vi "sub_ReadInput.vi"(8 "error in (no error)":errorcluster, 10 "Dynamic data":T1, 11 "Input parameters":T2={"Measurement type"=enum."Test", "Sensor type"=enum."HPK_8in_256", "Identifier"="test.txt", "Open after execution?"=FALSE, "Plot after execution?"=FALSE, "Display channel"=0, "Voltage Delay (s)"=0.5, "Switch Delay (s)"=0.01, "VISA resource name source"="", "VISA resource name DMM"="", "VISA resource name LCR"="", "Compliance  Level (uA)"=10.0, "Voltage Limit (V)"=1000.0, "Data storage location"="", "Scan voltages"="", "Use source as DMM?"=FALSE, "Single channel?"=FALSE, "LCR signal frequenzy (Hz)"=10.0} {"Voltage Limit (V)" format="%#_13g"; "Voltage Delay (s)" format="%#_13g"; "Switch Delay (s)" format="%#_13g"}) -> (0 "error out":errorcluster, 2 "Dynamic data":T1, 3 "Input parameters":T2={"Measurement type"=enum."Test", "Sensor type"=enum."HPK_8in_256", "Identifier"="test.txt", "Open after execution?"=FALSE, "Plot after execution?"=FALSE, "Display channel"=0, "Voltage Delay (s)"=0.5, "Switch Delay (s)"=0.01, "VISA resource name source"="", "VISA resource name DMM"="", "VISA resource name LCR"="", "Compliance  Level (uA)"=10.0, "Voltage Limit (V)"=1000.0, "Data storage location"="", "Scan voltages"="", "Use source as DMM?"=FALSE, "Single channel?"=FALSE, "LCR signal frequenzy (Hz)"=10.0} {"Voltage Limit (V)" format="%#_13g"; "Voltage Delay (s)" format="%#_13g"; "Switch Delay (s)" format="%#_13g"})   [LabVIEW 2016]
uses:
  Input_parameters.ctl
  Dynamic_data.ctl
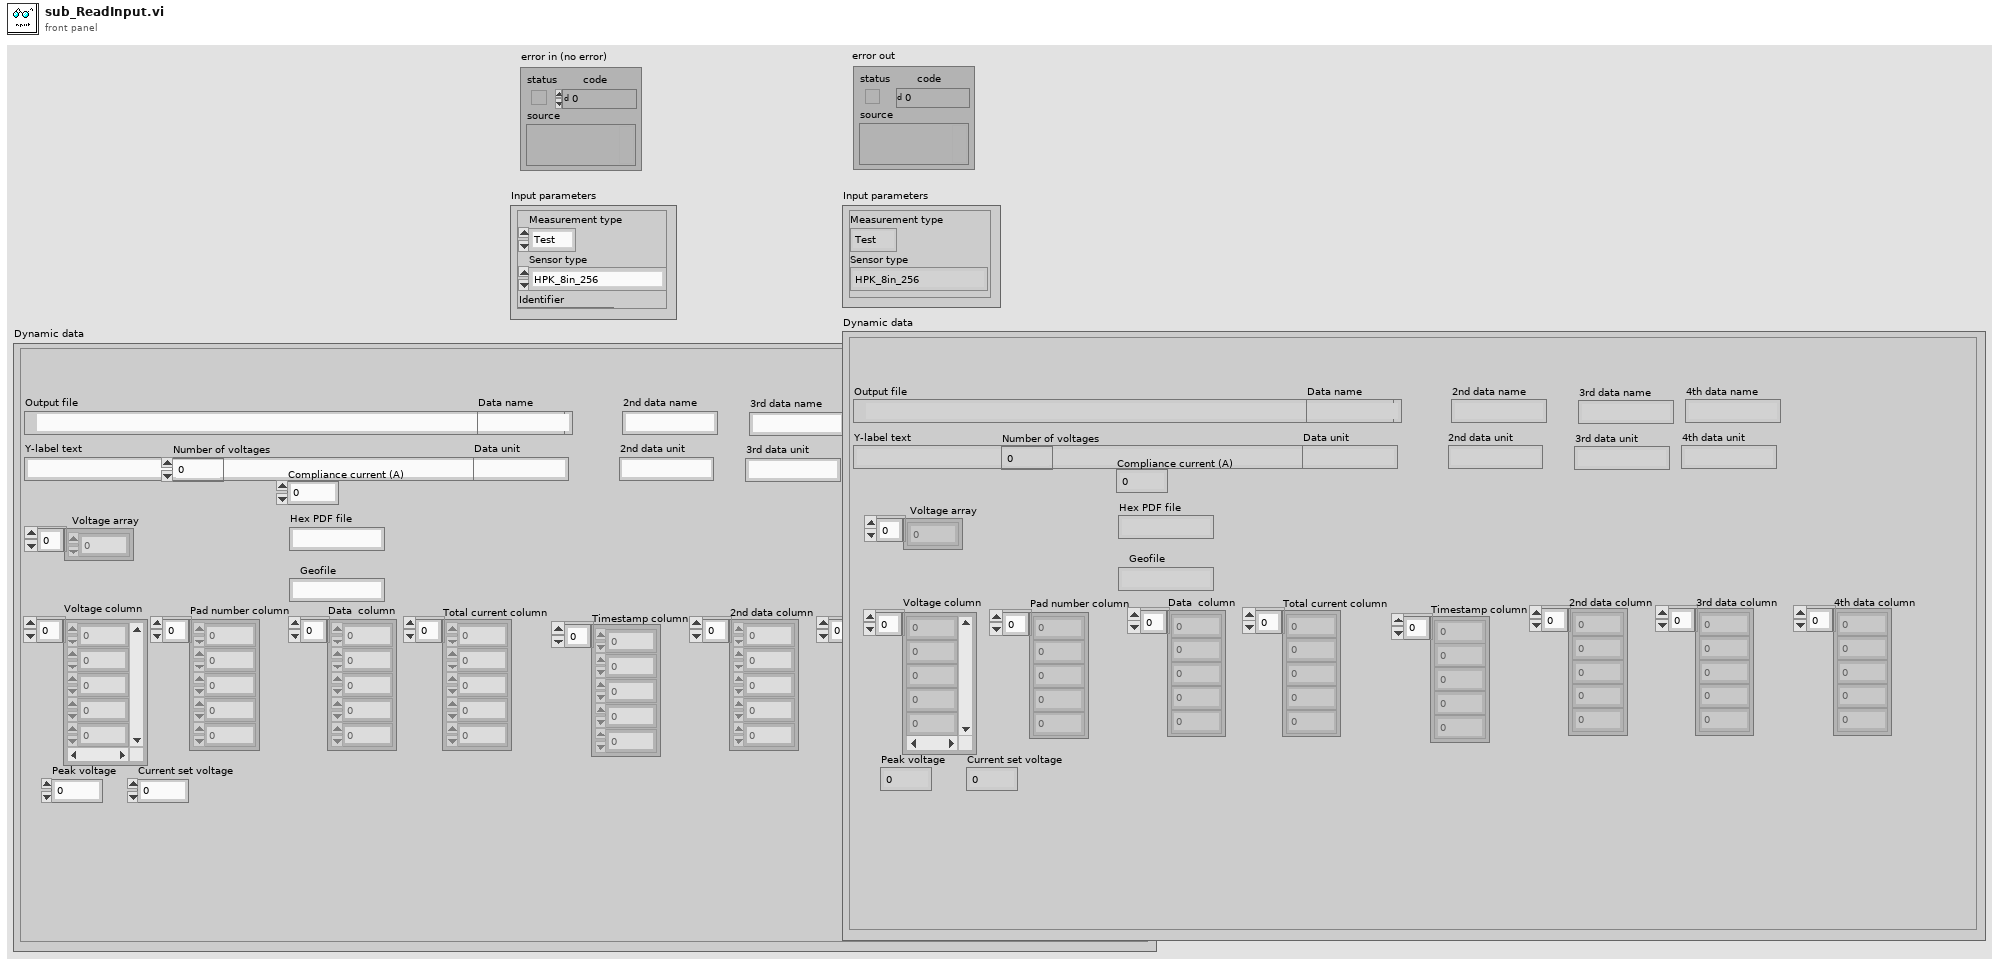
[diagram p1: front panel]
types:
  T1 = typedef "Dynamic_data.ctl" = cluster{"Output file":path, "Y-label text":string, "Current set voltage":dbl, "Voltage column":dbl[], "Pad number column":dbl[], "Data  column":dbl[], "Number of voltages":i32, "Compliance current (A)":dbl, "Geofile":string, "Peak voltage":dbl, "Hex PDF file":string, "Voltage array":dbl[], "Total current column":dbl[], "Timestamp column":dbl[], "Data name":string, "Data unit":string, "2nd data column":dbl[], "2nd data name":string, "2nd data unit":string, "3rd data column":dbl[], "4th data column":dbl[], "3rd data name":string, "3rd data unit":string, "4th data name":string, "4th data unit":string}
  T2 = typedef "Input_parameters.ctl" = cluster{"Measurement type":enum16{"IV", "CV", "Test"}, "Sensor type":enum16{"HPK_6in_135", "HPK_8in_256", "INF_8in_256", "Diode"}, "Identifier":string, "Open after execution?":bool, "Plot after execution?":bool, "Display channel":i32, "Voltage Delay (s)":dbl, "Switch Delay (s)":dbl, "VISA resource name source":refnum<visa-resource-name>, "VISA resource name DMM":refnum<visa-resource-name>, "VISA resource name LCR":refnum<visa-resource-name>, "Compliance  Level (uA)":dbl, "Voltage Limit (V)":dbl, "Data storage location":string, "Scan voltages":string, "Use source as DMM?":bool, "Single channel?":bool, "LCR signal frequenzy (Hz)":dbl}
  T3 = enum16{"HPK_6in_135", "HPK_8in_256", "INF_8in_256", "Diode"}
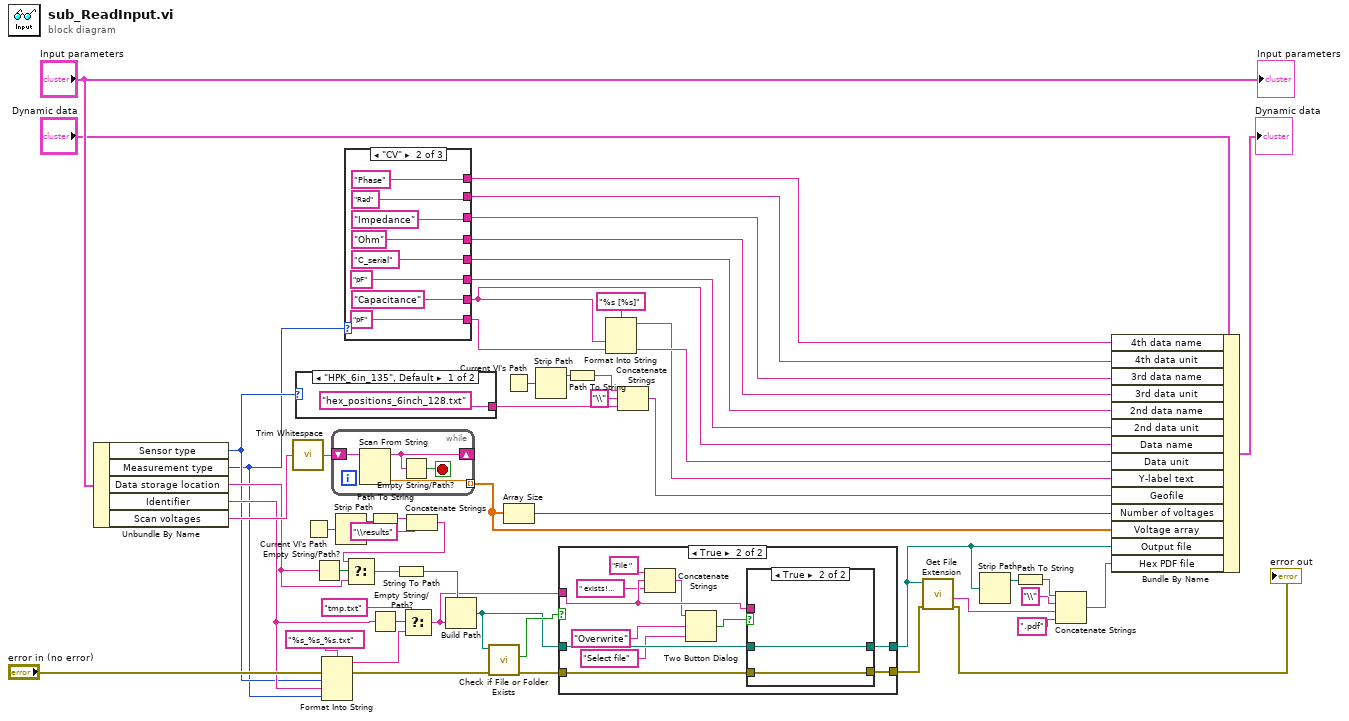
[diagram p0: block diagram]
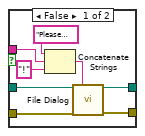
[diagram p3: hidden frame]
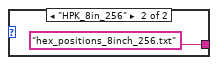
[diagram p4: hidden frame]
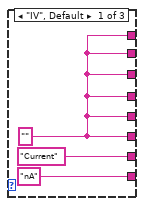
[diagram p5: hidden frame]
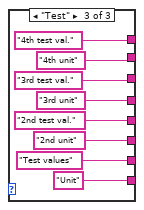
[diagram p6: hidden frame]
diagram:
  n1 = Unbundle By Name("Input parameters") -> ("Sensor type"=w20:T3, "Measurement type"=w19:enum16{"IV", "CV", "Test"}, "Data storage location"=w31:string, "Identifier"=w21:string, "Scan voltages"=w39:string)
  n2 = call <vilib>:"Trim Whitespace.vi"("string"=w39) -> ("trimmed string"=w40:string)  [unwired: 1 in]
  n3 = case shown="\"HPK_6in_135\", Default" w20 {
    tunnel: ["hex_positions_6inch_128.txt" "hex_positions_8inch_256.txt" ("name or relative path")] -> w51
    frame "HPK_6in_135", Default {
    }
    frame "HPK_8in_256" {
    }
  }
  n4 = Current VI's Path() -> (path=w35:path)
  n5 = Empty String/Path?(string/path=w31) -> (empty?=w36:bool)
  n6 = Format Into String(format string="%s_%s_%s.txt", error in="error in (no error)", w20, w21, w19) -> (resulting string=w23:string, error out=w13:errorcluster)  [unwired: 1 in]
  n7 = while {
    shift-right: [w58] -> _
    shift-left: w40 -> [w59]
    tunnel: [w60] -> w41 mode=indexing
    stop <- w57 stop-if-true
    n8 = Scan From String(input string=w59) -> (remaining string=w58:string, output 1=w60:dbl)  [unwired: 4 in, 2 out]
    n9 = Empty String/Path?(string/path=w58) -> (empty?=w57:bool)
  }
  n10 = Strip Path(path=w35) -> (stripped path=w34:path)  [unwired: 1 out]
  n11 = case shown="\"CV\"" w19 {
    tunnel: ["Current" "Capacitance" "Test values"] -> w9
    tunnel: ["nA" "pF" "Unit"] -> w10
    tunnel: [w61 "C_serial" "2nd test val."] -> w8
    tunnel: [w61 "pF" "2nd unit"] -> w7
    tunnel: [w61 "Ohm" "3rd unit"] -> w4
    tunnel: [w61 "Impedance" "3rd test val."] -> w3
    tunnel: [w61 "Rad" "4th unit"] -> w2
    tunnel: [w61 "Phase" "4th test val."] -> w1
    frame "IV", Default {
      w61 = ""
    }
    frame "CV" {
    }
    frame "Test" {
    }
  }
  n12 = Path To String(path=w34) -> (string=w33:string)
  n13 = Empty String/Path?(string/path=w21) -> (empty?=w27:bool)
  n14 = Select(t="tmp.txt", s=w27, f=w23) -> (s? t:f=w12:string)
  n15 = Concatenate Strings(w33, "\\results" ("string")) -> (w30:string)
  n16 = Select(t=w30, s=w36, f=w31) -> (s? t:f=w29:string)
  n17 = String To Path(string=w29) -> (path=w28:path)
  n18 = Build Path(base path=w28, name or relative path=w12) -> (appended path=w17:path)
  n19 = call <vilib>:"Check if File or Folder Exists.vi"("error in (no error)"=w13, "path"=w17) -> ("error out"=w15:errorcluster, "file or folder exists?"=w18:bool)  [unwired: 7 in, 1 out]
  n20 = Current VI's Path() -> (path=w38:path)
  n21 = Array Size(array=w41) -> (size(s)=w42:i32)
  n22 = Strip Path(path=w38) -> (stripped path=w37:path)  [unwired: 1 out]
  n23 = case shown="True" w18 {
    tunnel: w17 -> [w81 w92]
    tunnel: [w81 w91] -> w16
    tunnel: w15 -> [w80 w90]
    tunnel: [w80 w89] -> w14
    tunnel: w12 -> [_ w88]
    frame False {
    }
    frame True {
      n24 = Concatenate Strings("File " ("string"), w88, " exists! Overwite?" ("string")) -> (w85:string)
      n25 = Two Button Dialog(message=w85, 1:"Select file" ("Center Button Text (\"No\")"), 2:"Overwrite" ("Left Button Text (\"Yes\")")) -> (T button?=w82:bool)
      n26 = case shown="True" w82 {
        tunnel: w92 -> [w100 w102]
        tunnel: [w99 w102] -> w91
        tunnel: w90 -> [w98 w101]
        tunnel: [w97 w101] -> w89
        tunnel: w88 -> [w94 _]
        frame False {
          n27 = Concatenate Strings("Please chose a new file instead of  " ("prompt (Choose or enter file path)"), w94, "!" ("string")) -> (w96:string)
          n28 = call "File Dialog"("start path"=w100, "prompt"=w96, "error in"=w98) -> ("selected path"=w99:path, "error out"=w97:errorcluster)  [unwired: 9 in, 2 out]
        }
        frame True {
        }
      }
    }
  }
  n29 = Path To String(path=w37) -> (string=w25:string)
  n30 = Format Into String(format string="%s [%s]", w9, w10) -> (resulting string=w5:string)  [unwired: 2 in, 1 out]
  n31 = Concatenate Strings(w25, "\\" ("string"), w51) -> (w6:string)
  n32 = call <vilib>:"Get File Extension.vi"("error in (no error)"=w14, "file"=w16) -> ("error out"=→"error out":errorcluster, "filename without extension"=w48:string)  [unwired: 5 in, 3 out]
  n33 = Strip Path(path=w16) -> (stripped path=w46:path)  [unwired: 1 out]
  n34 = Path To String(path=w46) -> (string=w45:string)
  n35 = Concatenate Strings(w45, "\\" ("string"), w48, ".pdf" ("string")) -> (w49:string)
  n36 = Bundle By Name(cluster="Dynamic data", "4th data name"=w1, "4th data unit"=w2, "3rd data name"=w3, "3rd data unit"=w4, "2nd data name"=w8, "2nd data unit"=w7, "Data name"=w9, "Data unit"=w10, "Y-label text"=w5, "Geofile"=w6, "Number of voltages"=w42, "Voltage array"=w41, "Output file"=w16, "Hex PDF file"=w49) -> (→"Dynamic data":T1)
  "Input parameters" <- "Input parameters"
